vi "Init.vi"(8 "error in (no error)":errorcluster, 9 "Config File Path":path=path "", 10 "Name":string, 11 "Process In":refnum<class "Debug Message Receiver.lvclass">) -> (0 "error out":errorcluster, 3 "Process Out":refnum<class "Debug Message Receiver.lvclass">)   [LabVIEW 2020, in "Debug Message Receiver.lvclass"]
doc: "Initializes the process and creates necessary references. Anything initialized here is released in the Clear.vi method."
uses:
  Debug Message Receiver.lvclass
  Debug Message Receiver.lvclass/Debug Message Receiver.ctl
  Process/Debug Process.lvclass
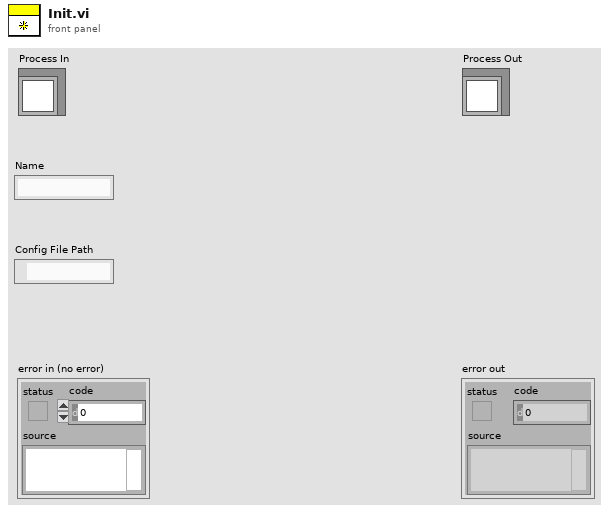
[diagram p1: front panel]
types:
  T1 = cluster{"Action":string, "Call Chain":string, "Process":string, "Message":string, "Message Data":variant, "Time":u32}
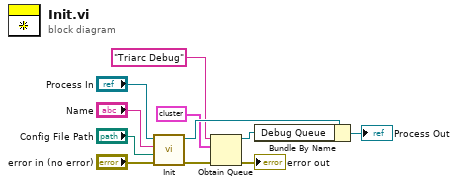
[diagram p0: block diagram]
diagram:
  n1 = call-parent "Init.vi"("error in (no error)"="error in (no error)", "Config File Path"="Config File Path", "Name"="Name", "Process In"="Process In") -> ("error out"=w3:errorcluster, "Process Out"=w11:refnum<class "Debug Message Receiver.lvclass">)  [unwired: 6 in]
  n2 = Obtain Queue(name (unnamed)="Triarc Debug", element data type=T1 {"Action"="", "Call Chain"="", "Process"="", "Message"="", "Message Data"=variant, "Time"=0} ("output cluster"), error in (no error)=w3) -> (queue out=w1:refnum<queue>, error out=→"error out":errorcluster)  [unwired: 2 in, 1 out]
  n3 = Bundle By Name(cluster=w11, "Debug Queue"=w1) -> (→"Process Out":refnum<class "Debug Message Receiver.lvclass">)
